vi "frw_round_2Darraysize.vi"(10 "block size":i32=1, 11 "array in":dbl[][](array[numeric])) -> (0 "nBlocks":i32, 1 "nCol":i32, 2 "nRows":i32, 3 "array out":dbl[][](array[numeric]))   [LabVIEW 2013]
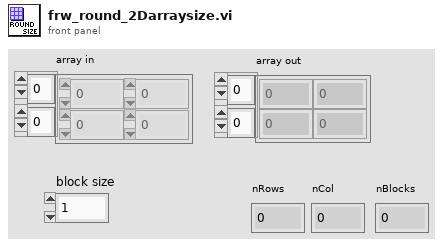
[diagram p1: front panel]
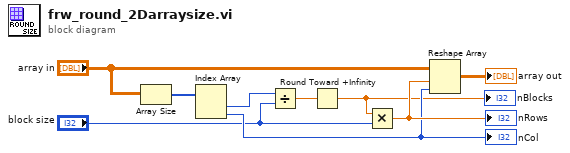
[diagram p0: block diagram]
diagram:
  n1 = Array Size(array="array in") -> (size(s)=w9:i32[])
  n2 = Index Array(array=w9) -> (element #1=w6:i32, element #2=w7:i32)  [unwired: 2 in]
  "nCol" <- w7
  n3 = Divide(x=w6, y="block size") -> (x/y=w4:dbl)
  n4 = Round Toward +Infinity(x=w4) -> (ceil(x): smallest int >= x=w3:dbl)
  "nBlocks" <- w3
  n5 = Multiply(x=w3, y="block size") -> (x*y=w8:dbl)
  "nRows" <- w8
  n6 = Reshape Array("array in", w8, w7) -> (→"array out":dbl[][])
